vi "get supported types.vi"(8 "error in":errorcluster, 11 "user tag bus module configuration In":refnum<class "fixed channel tag bus module configuration.lvclass">) -> (0 "error out":errorcluster, 2 "supported types":T1[](array[typedef]), 3 "user tag bus module configuration Out":refnum<class "fixed channel tag bus module configuration.lvclass">)   [LabVIEW 2013, in "fixed channel tag bus module configuration.lvclass"]
doc: "Provides an interface for determining the targets supported by a given configuration/runtime class pairing. This should be overridden by any useful child class."
uses:
  fixed channel tag bus module configuration.lvclass
  <vilib>/NI/Tag Bus/tag/Data Type.ctl
  fixed channel tag bus module configuration.lvclass/fixed channel tag bus module configuration.ctl
  <vilib>/NI/Tag Bus/tag/tag descriptor.lvclass/tag descriptor.ctl
  <vilib>/NI/Tag Bus/tag/tag descriptor.lvclass
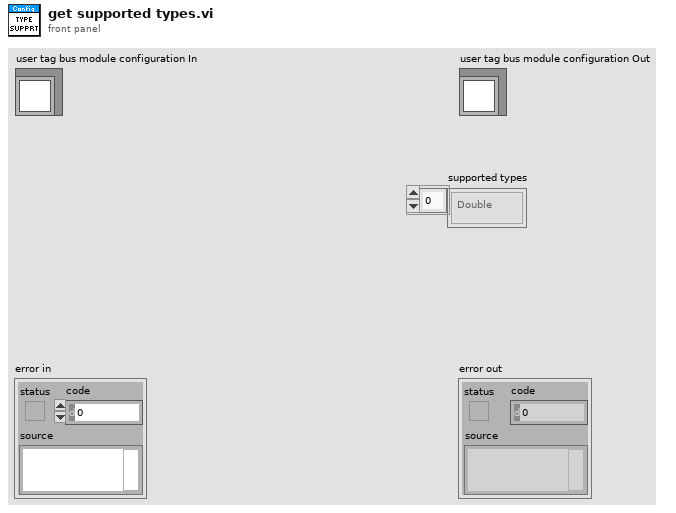
[diagram p1: front panel]
types:
  T1 = typedef "tag bus.lvlib/tag descriptor.lvclass/Data Type.ctl" = enum16{"Double", "Single", "I64", "I32", "I16", "I8", "U64", "U32", "U16", "U8", "Boolean", "String", "Array of Double", "Array of Single", "Array of I64", "Array of I32", "Array of I16", "Array of I8", "Array of U64", "Array of U32", "Array of U16", "Array of U8", "Array of Boolean", "Array of String"}
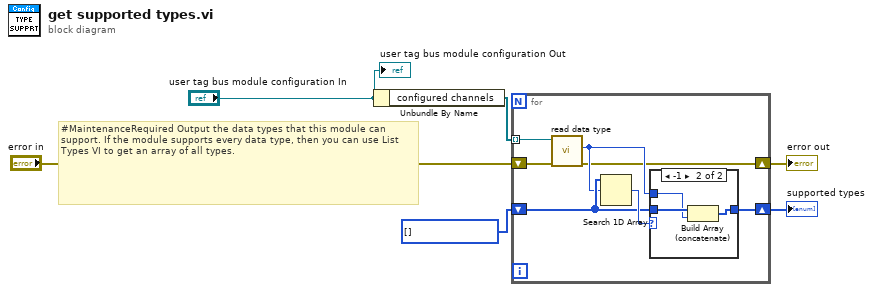
[diagram p0: block diagram]
diagram:
  w4 = T1[] [] items=["Double", "Single", "I64", "I32", "I16", "I8", "U64", "U32", "U16", "U8", "Boolean", "String", "Array of Double", "Array of Single", "Array of I64", "Array of I32", "Array of I16", "Array of I8", "Array of U64", "Array of U32", "Array of U16", "Array of U8", "Array of Boolean", "Array of String"]
  # "#MaintenanceRequired Output the data types that this module can support. If the module supports every data type, then you can use List Types VI to get an array of all types."
  n1 = Unbundle By Name("user tag bus module configuration In") -> ("configured channels"=w5:refnum<class "TBM channel.lvclass">[])
  n2 = for {
    tunnel: w5 -> [w13] mode=indexing
    shift-right: [w9] -> w3
    shift-left: w4 -> [w11]
    shift-right: [w7] -> w1
    shift-left: "error in" -> [w8]
    n3 = call <vilib>:"read data type.vi"("error in"=w8, "system tag in"=w13) -> ("error out"=w7:errorcluster, "data type"=w10:T1)  [unwired: 7 in, 1 out]
    n4 = Search 1D Array(1D array=w11, element=w10) -> (index of element=w12:i32)  [unwired: 1 in]
    n5 = case shown="-1" w12 {
      tunnel: w11 -> [w14 w17]
      tunnel: w10 -> [_ w16]
      tunnel: [w14 w15] -> w9
      frame Default {
      }
      frame -1 {
        n6 = Build Array (concatenate)(w17, w16) -> (w15:T1[])
      }
    }
  }
  "error out" <- w1
  "supported types" <- w3
  "user tag bus module configuration Out" <- "user tag bus module configuration In"
